vi "ForLoop_subIf.vi"() -> ()   [LabVIEW 2018]
panel:
  out "배열":i32[](array[numeric])
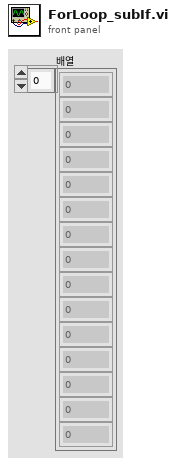
[diagram p1: front panel]
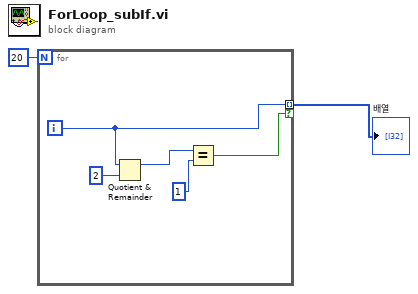
[diagram p0: block diagram]
diagram:
  n1 = for {
    N: 20 -> [_]
    tunnel: [w4] -> w2 mode=indexing if=w3
    i -> [w4]
    n2 = Quotient & Remainder(x=w4, y=2) -> (x-y*floor(x/y)=w6:i32)  [unwired: 1 out]
    n3 = Equal?(x=w6, y=1) -> (x = y?=w3:bool)
  }
  "배열" <- w2
